vi "Read Discriminator Level (Scan).vi"(8 "error in (no error)":errorcluster, 10 "Discriminator (A)":T1, 11 "VISA resource name":refnum<visa-resource-name>) -> (0 "error out":errorcluster, 1 "Discriminator Level":dbl=0.01 format="%.4g", 3 "VISA resource name out":refnum<visa-resource-name>)   [LabVIEW 2013, in "SRS SR400.lvlib"]
doc: "<B>DZ i</B>\n\nThe DZ command returns the level of discriminator i during a scan. i = 0,1, or 2 designates discriminator A B, or T and is required. If discriminator i is in the SCAN mode, its current level during a scan is read. If the counters are in reset or the discriminator is in the FIXED mode, the DZ command returns the starting value for the level (same as DL command). The DZ command is a read only command."
uses:
  <instrlib>/SRS SR400/SRS SR400.lvlib
  <instrlib>/SRS SR400/Public/Typedefs/Discriminator.ctl
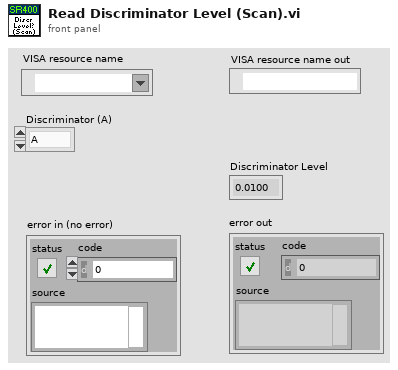
[diagram p1: front panel]
types:
  T1 = typedef "SRS SR400.lvlib/Discriminator.ctl" = enum16{"A", "B", "T"}
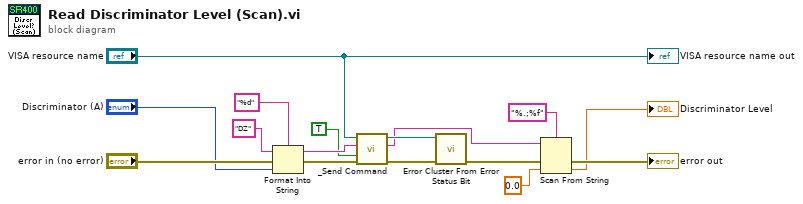
[diagram p0: block diagram]
diagram:
  n1 = Format Into String(format string="%d", initial string="DZ" ("command"), error in="error in (no error)", "Discriminator (A)") -> (resulting string=w9:string, error out=w8:errorcluster)
  n2 = call <instrlib>:"_Send Command.vi"("error in (no error)"=w8, "Read Value? (F)"=TRUE, "Command"=w9, "VISA resource name"="VISA resource name") -> ("error out"=w4:errorcluster, "Response"=w2:string, "VISA resource name out"=w5:refnum<visa-resource-name>)  [unwired: 5 out]
  n3 = call <instrlib>:"Error Cluster From Error Status Bit.vi"("error in (no error)"=w4, "VISA resource name"=w5) -> ("error out"=w3:errorcluster)  [unwired: 8 in, 1 out]
  n4 = Scan From String(format string="%.;%f", input string=w2, error in=w3, default 1=0.0 ("default value 1")) -> (error out=→"error out":errorcluster, output 1=→"Discriminator Level":dbl)  [unwired: 1 in, 2 out]
  "VISA resource name out" <- "VISA resource name"
